vi "例13.2 仿真信号的生成子程序.vi"(3 "信噪比":dbl=1.0 format="%.2p", 4 "sampling info":cluster{"Fs":dbl, "#s":dbl}={"Fs"=1000.0, "#s"=1000.0} caption="采样信息" {"Fs" format="%.2p"}, 5 "square wave \nduty cycle (%)":dbl=50.0 caption="方波占空比(%)" format="%0.2f", 6 "formula":string="sin(w*t)*sin(2*pi(1)*t)" caption="公式", 7 "相位":dbl, 8 "幅值":dbl, 9 "频率":dbl, 10 "噪声选择":enum16{"无", "均匀白噪声", "高斯噪声"}(ring), 11 "波形选择":enum16{"正弦波", "三角波", "方波", "公式波"}(ring)) -> (1 "波形图":waveform(dbl)(graph))   [LabVIEW 2012]
uses:
  <vilib>/measure/NI_MABase.lvlib
  <vilib>/measure/NI_MAPro.lvlib
panel:
  # "波 形 发 生 器"
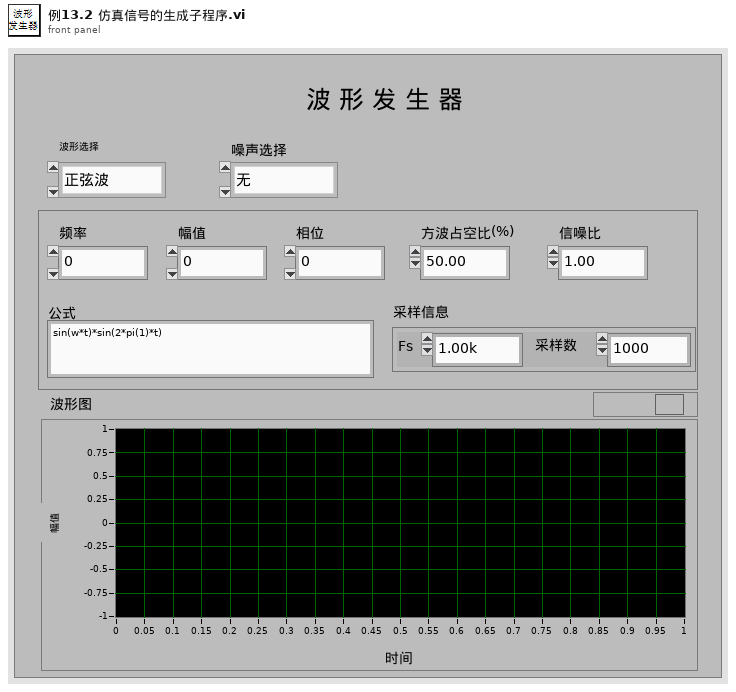
[diagram p1: front panel]
types:
  T1 = enum16{"Sine Wave", "Triangle Wave", "Square Wave", "Sawtooth Wave"}
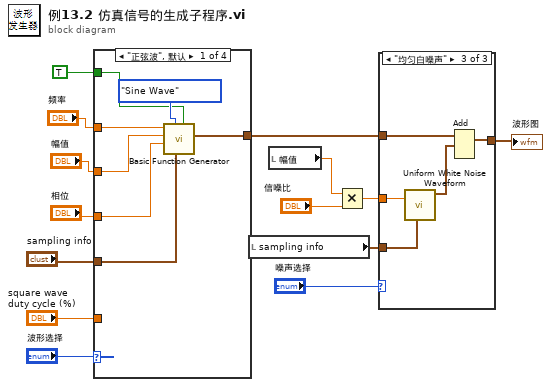
[diagram p0: block diagram]
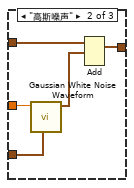
[diagram p3: hidden frame]
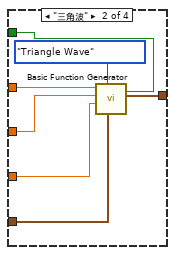
[diagram p4: hidden frame]
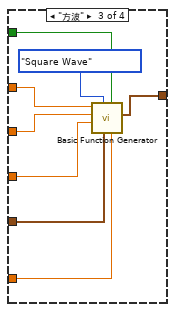
[diagram p5: hidden frame]
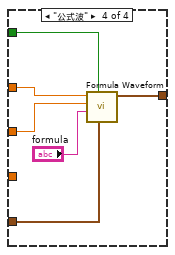
[diagram p6: hidden frame]
diagram:
  n1 = case shown="\"正弦波\", 默认" "波形选择" {
    tunnel: [w17 w28 w30 w39] -> w12
    tunnel: "频率" -> [w20 w26 w35 w42]
    tunnel: "幅值" -> [w19 w25 w34 w41]
    tunnel: "相位" -> [w16 w24 w33 _]
    tunnel: "sampling info" -> [w18 w23 w32 w38]
    tunnel: "square wave \nduty cycle (%)" -> [_ _ w31 _]
    tunnel: TRUE ("reset signal") -> [w15 w22 w29 w37]
    frame "正弦波", Default {
      n2 = call <vilib>:"Basic Function Generator.vi"("reset signal"=w15, "sampling info"=w18, "signal type"=T1."Sine Wave", "phase"=w16, "amplitude"=w19, "frequency"=w20) -> ("signal out"=w17:waveform(dbl))  [unwired: 3 in, 2 out]
    }
    frame "三角波" {
      n3 = call <vilib>:"Basic Function Generator.vi"("reset signal"=w22, "sampling info"=w23, "signal type"=T1."Triangle Wave", "phase"=w24, "amplitude"=w25, "frequency"=w26) -> ("signal out"=w28:waveform(dbl))  [unwired: 3 in, 2 out]
    }
    frame "方波" {
      n4 = call <vilib>:"Basic Function Generator.vi"("square wave duty cycle (%)"=w31, "reset signal"=w29, "sampling info"=w32, "signal type"=T1."Square Wave", "phase"=w33, "amplitude"=w34, "frequency"=w35) -> ("signal out"=w30:waveform(dbl))  [unwired: 2 in, 2 out]
    }
    frame "公式波" {
      n5 = call <vilib>:"Formula Waveform.vi"("sampling info"=w38, "reset signal"=w37, "formula"="formula", "amplitude"=w41, "frequency"=w42) -> ("signal out"=w39:waveform(dbl))  [unwired: 5 in, 1 out]
    }
  }
  n6 = local read "sampling info"() -> (w4:cluster{"Fs":dbl, "#s":dbl})
  n7 = local read "幅值"() -> (w13:dbl)
  n8 = Multiply(x=w13, y="信噪比") -> (x*y=w11:dbl)
  n9 = case shown="\"均匀白噪声\"" "噪声选择" {
    tunnel: [w43 w47 w50] -> w1
    tunnel: w11 -> [_ w48 w53]
    tunnel: w12 -> [w43 w46 w52]
    tunnel: w4 -> [_ w45 w49]
    frame "无", Default {
    }
    frame "高斯噪声" {
      n10 = call <vilib>:"Gaussian White Noise Waveform.vi"("sampling info"=w45, "standard deviation"=w48) -> ("signal out"=w44:waveform(dbl))  [unwired: 8 in, 1 out]
      n11 = Add(1:w44, 2:w46) -> (0:w47:waveform(dbl))  [unwired: 1 in, 1 out]
    }
    frame "均匀白噪声" {
      n12 = call <vilib>:"Uniform White Noise Waveform.vi"("sampling info"=w49, "amplitude"=w53) -> ("signal out"=w51:waveform(dbl))  [unwired: 8 in, 1 out]
      n13 = Add(1:w51, 2:w52) -> (0:w50:waveform(dbl))  [unwired: 1 in, 1 out]
    }
  }
  "波形图" <- w1
